vi "Append to Array - Object.vi"(8 "error in (no error)":errorcluster, 10 "JSON Object":variant, 11 "JSON Tree in (JSON Array)":variant) -> (0 "error out":errorcluster, 3 "JSON Tree out (JSON Array)":variant)   [LabVIEW 2015, in "i3-json.lvlib"]
doc: "Use this template to build a VI to use as a subVI."
uses:
  i3-json.lvlib
  JSON Types/JSON Type.ctl
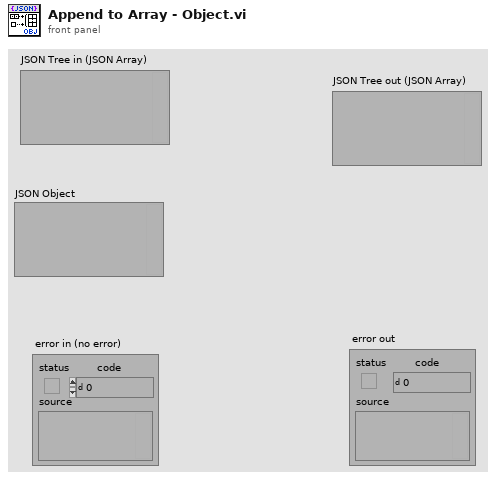
[diagram p1: front panel]
types:
  T1 = typedef "i3-json.lvlib/JSON Type.ctl" = enum8{"JSON Compatible", "JSON Array", "JSON Object", "JSON Null", "Double", "String", "Boolean", "Unknown"}
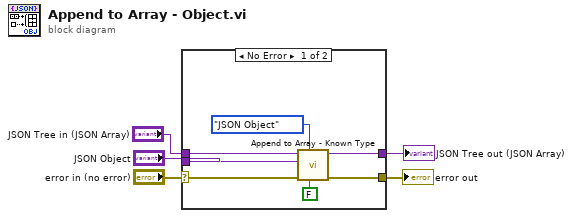
[diagram p0: block diagram]
diagram:
  n1 = case shown="No Error" "error in (no error)" {
    selector: "error in (no error)" -> [w10 w14]
    tunnel: [w11 w14] -> w4
    tunnel: [w12 w13] -> w3
    tunnel: "JSON Tree in (JSON Array)" -> [w9 w13]
    tunnel: "JSON Object" -> [w8 _]
    frame No Error {
      n2 = call "Append to Array - Known Type.vi"("Add Parameter as JSON Tree?"=FALSE, "JSON Type"=JSON_Type."JSON Object", "error in (no error)"=w10, "Value"=w8, "JSON Tree in (JSON Array)"=w9) -> ("error out"=w11:errorcluster, "JSON Tree out (JSON Array)"=w12:variant)  [unwired: 5 in]
    }
    frame Error {
    }
  }
  "error out" <- w4
  "JSON Tree out (JSON Array)" <- w3
